vi "BMark_Save Tokens.vi"(10 "reference":refnum<vi>, 11 "GroupByVI":bool) -> ()   [LabVIEW 2018, in "Bookmark Manager.lvlib"]
uses:
  Bookmark Manager.lvlib
  <resource>/dialog/lvconfig.llb/LV Config Write String.vi
  <resource>/dialog/lvconfig.llb/LV Config Write Boolean.vi
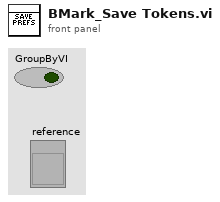
[diagram p1: front panel]
types:
  T1 = typedef "LVRectTypeDef.ctl" = cluster{"Left":i16, "Top":i16, "Right":i16, "Bottom":i16}
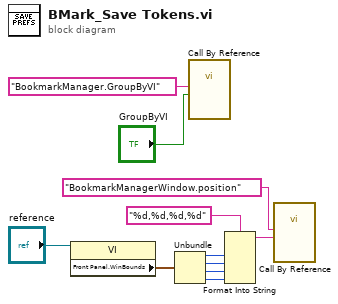
[diagram p0: block diagram]
diagram:
  n1 = property class="VI"(reference="reference") -> ("Front Panel.WinBounds"=w10:T1)  [unwired: 1 in, 2 out]
  n2 = Unbundle(w10) -> ("Left"=w4:i16, "Top"=w5:i16, "Right"=w6:i16, "Bottom"=w7:i16)
  n3 = call-by-ref "?"("value"="GroupByVI", "key"="BookmarkManager.GroupByVI") -> ()  [unwired: 7 in, 3 out]
  n4 = Format Into String(format string="%d,%d,%d,%d", w4, w5, w6, w7) -> (resulting string=w9:string)  [unwired: 2 in, 1 out]
  n5 = call-by-ref "?"("value"=w9, "key"="BookmarkManagerWindow.position") -> ()  [unwired: 3 in, 7 out]
